vi "ex5_sharedlog.vi"() -> ()   [LabVIEW 2022 SP3]
uses:
  C:/Program Files (x86)/National Instruments/LabVIEW 2022/examples/Connectivity/Python/support/PythonVersionsEnum.ctl
  py_msg.ctl
  pylabview/pythonq.lvlib
panel:
  out "String":string
  out "xref out":string
  out "Data Out":dbl(graph)
  out "xref in":string
  in  "wait":u32=500
  out "Data IN":dbl(graph)
  in  "stop":bool
  # "https://github.com/jmor2000/labview_python_bridge"
  # "brought to you by"
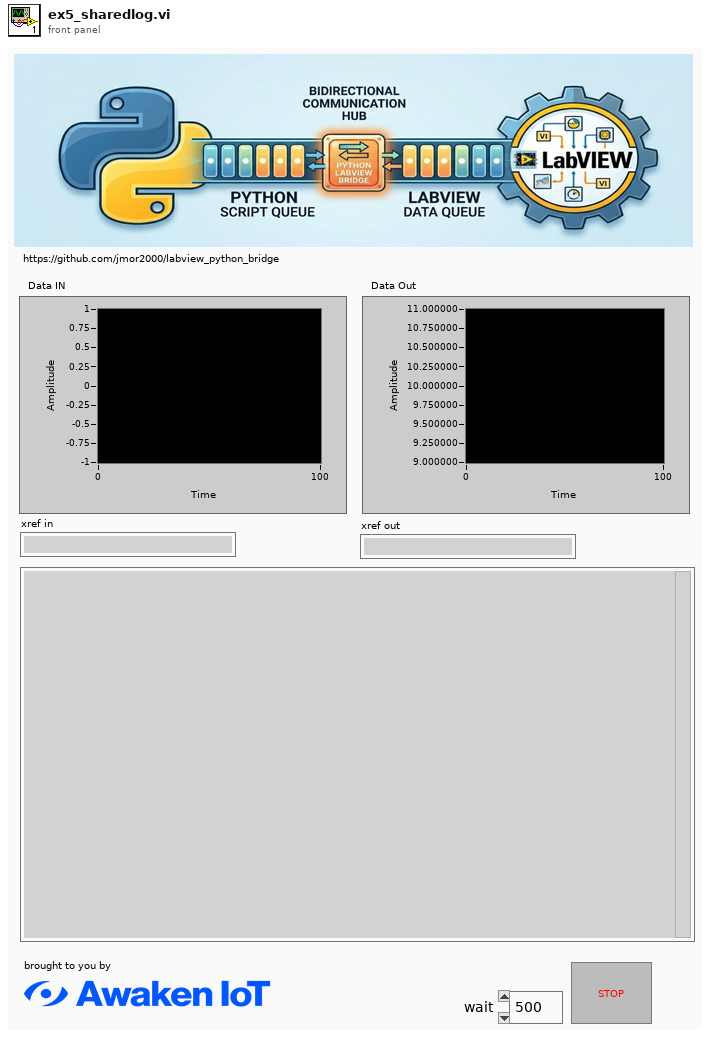
[diagram p1: front panel]
types:
  T1 = typedef "PythonVersionsEnum.ctl" = enum16{"3.6", "3.7", "3.8", "3.9"}
  T2 = typedef "pythonq.lvlib/py_cluster.ctl" = cluster{"path":path, "py":T3}
  T3 = typedef "pythonq.lvlib/py_session.ctl" = cluster{"session":refnum<k35>, "object":refnum<k38>}
  T4 = cluster{"id":string, "ts":string, "msg":string, "iref":string, "xref":string}
  T5 = typedef "pythonq.lvlib/py_result.ctl" = cluster{"value":string, "ok":bool, "error_msg":string}
  T6 = typedef "py_msg.ctl" = cluster{"double":dbl, "ref":string}
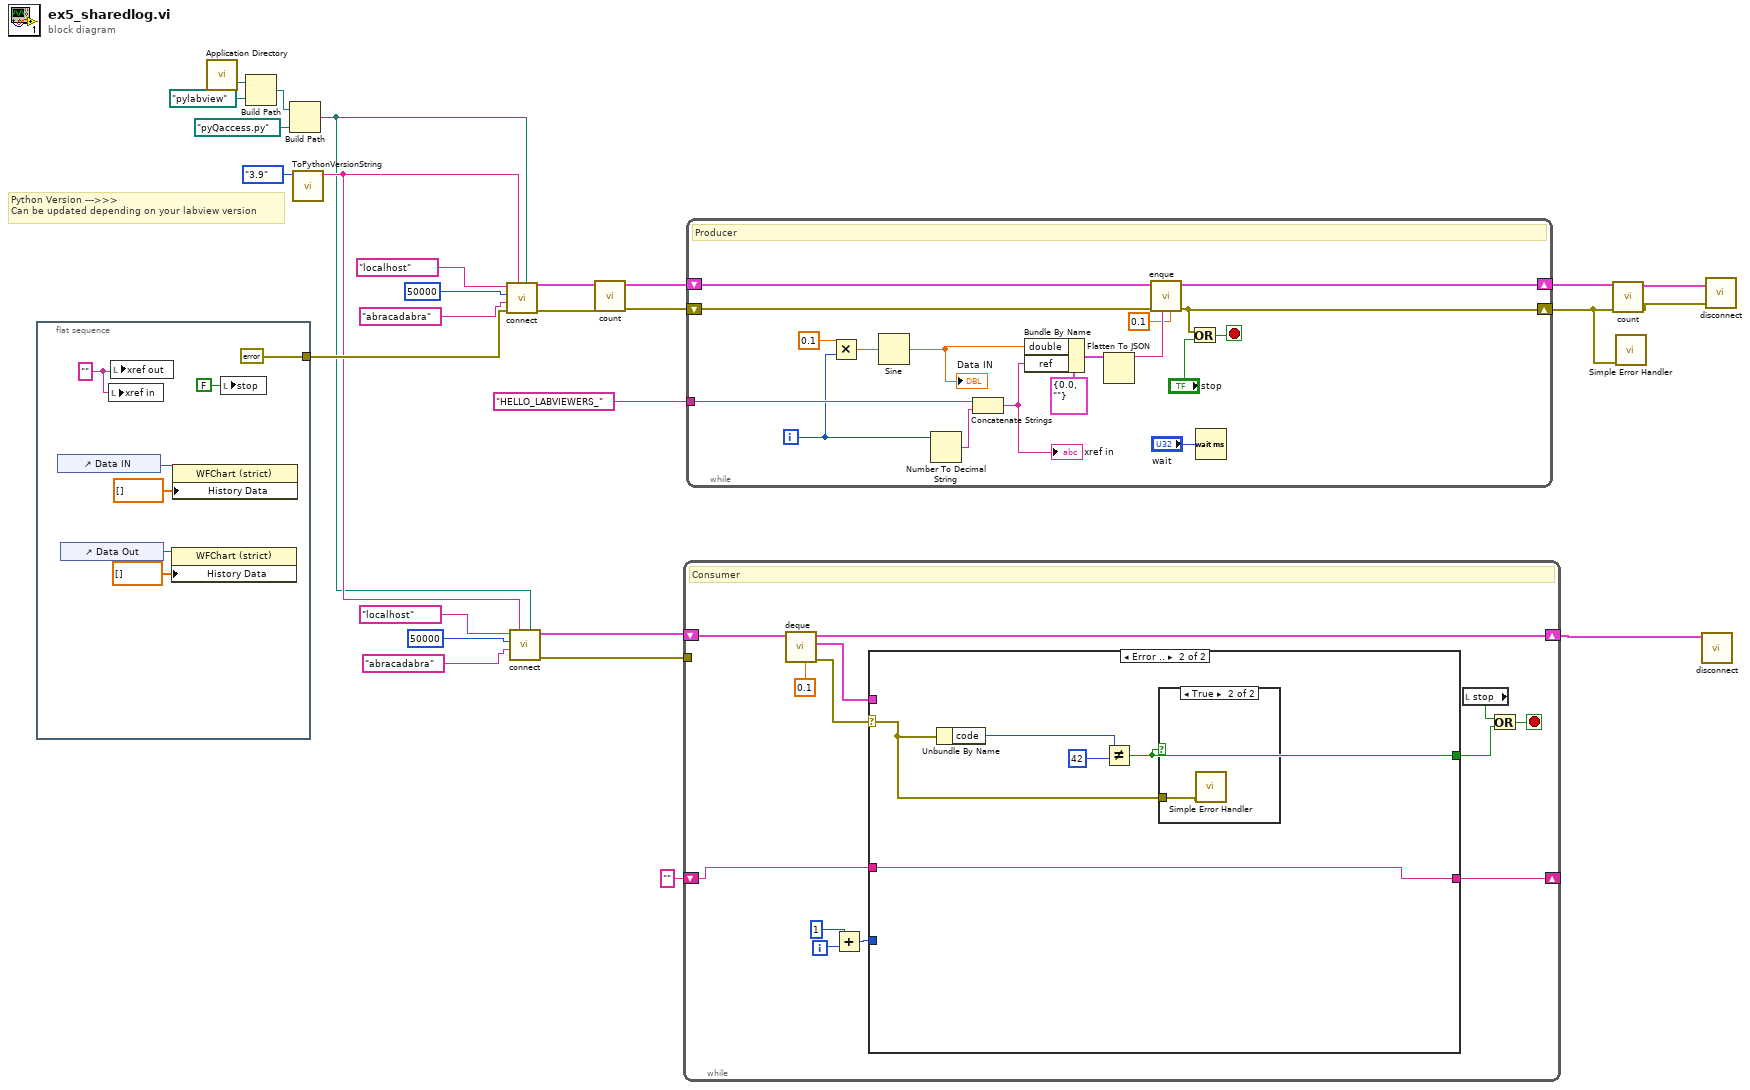
[diagram p0: block diagram]
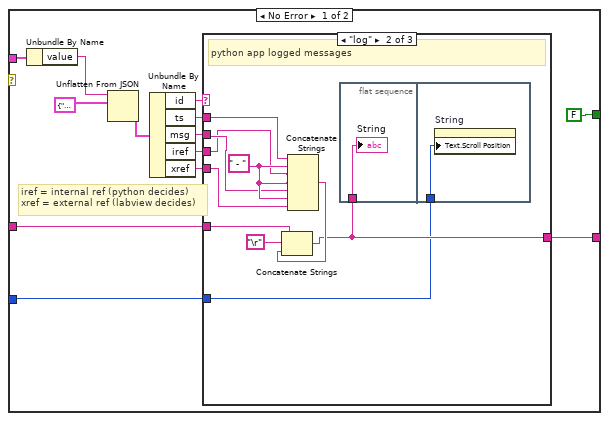
[diagram p2: hidden frame]
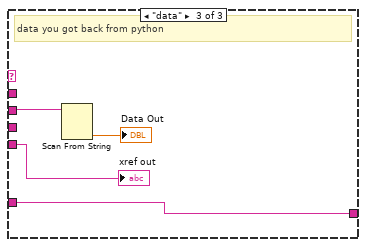
[diagram p4: hidden frame]
diagram:
  # "Python Version --->>>\nCan be updated depending on your labview version"
  n1 = flat-sequence {
    tunnel: [errorcluster {"status"=FALSE, "code"=0, "source"=""} ("error in (no error)")] -> w16
    frame #0 {
      w30 = "" ("cur ref 2")
      n2 = control-ref of="Data IN"() -> (w32:refnum<vi>)
      n3 = control-ref of="Data Out"() -> (w29:refnum<vi>)
      n4 = local write "xref in"(w30) -> ()
      n5 = local write "xref out"(w30) -> ()
      n6 = property class="WFChart (strict)"(reference=w29, "History Data"=dbl[] []) -> ()  [unwired: 1 in, 2 out]
      n7 = property class="WFChart (strict)"(reference=w32, "History Data"=dbl[] []) -> ()  [unwired: 1 in, 2 out]
      n8 = local write "stop"(FALSE ("stop")) -> ()
    }
  }
  n9 = call <vilib>:"Application Directory.vi"() -> ("Application Directory"=w22:path)
  n10 = Build Path(base path=w22, name or relative path=path "pylabview") -> (appended path=w23:path)
  n11 = Build Path(base path=w23, name or relative path=path "pyQaccess.py") -> (appended path=w7:path)
  n12 = call "ToPythonVersionString.vi"("python version"=PythonVersionsEnum."3.9") -> ("python version string"=w8:string)  [unwired: 10 in]
  n13 = call "connect.vi"("module path"=w7, "Python version"=w8, "error in (no error)"=w16, "password"="abracadabra", "port"=50000, "ip_address"="localhost") -> ("error out"=w18:errorcluster, "py out"=w17:T2)  [unwired: 4 in]
  n14 = call "connect.vi"("module path"=w7, "Python version"=w8, "password"="abracadabra", "port"=50000, "ip_address"="localhost") -> ("error out"=w5:errorcluster, "py out"=w6:T2)  [unwired: 5 in]
  n15 = call "count.vi"("error in (no error)"=w18, "py in"=w17) -> ("error out"=w15:errorcluster, "py out"=w12:T2)  [unwired: 7 in, 1 out]
  n16 = while {
    shift-right: [w46] -> w3
    shift-left: w6 -> [w47]
    tunnel: w5 -> [_]
    shift-right: [w38] -> _
    shift-left: "" -> [w39]
    i -> [w37]
    stop <- w43 stop-if-true
    # "Consumer"
    n17 = call "deque.vi"("timeout"=0.1, "py in"=w47) -> ("error out"=w44:errorcluster, "response"=w41:T5, "py out"=w46:T2)  [unwired: 6 in, 1 out]
    n18 = Add(x=1, y=w37) -> (x+y=w35:i32)
    n19 = case shown="Error .." w44 {
      selector: w44 -> [_ w78]
      tunnel: [FALSE w79] -> w42
      tunnel: w41 -> [w59 _]
      tunnel: [w50 w80] -> w38
      tunnel: w39 -> [w49 w80]
      tunnel: w35 -> [w48 _]
      frame No Error {
        # "iref = internal ref (python decides)\nxref = external ref (labview decides)"
        n20 = Unbundle By Name(w59) -> ("value"=w58:string)
        n21 = Unflatten From JSON(JSON string=w58, type and defaults=T4 {"id"="", "ts"="", "msg"="", "iref"="", "xref"=""}) -> (value=w57:T4)  [unwired: 5 in, 1 out]
        n22 = Unbundle By Name(w57) -> ("id"=w55:string, "ts"=w54:string, "msg"=w53:string, "iref"=w52:string, "xref"=w51:string)
        n23 = case shown="\"log\"" w55 {
          tunnel: w54 -> [_ w71 _]
          tunnel: w53 -> [_ w63 w77]
          tunnel: w52 -> [_ w62 _]
          tunnel: w51 -> [_ w67 w75]
          tunnel: [w61 w65 w74] -> w50
          tunnel: w49 -> [w61 w68 w74]
          tunnel: w48 -> [_ w64 _]
          frame "", Default {
            # "Unknown msg type"
          }
          frame "log" {
            w66 = " - "
            # "python app logged messages"
            n24 = Concatenate Strings(w71, w66, w62, w66, w63, w66, w67) -> (w69:string)
            n25 = Concatenate Strings(w68, "\r", w69) -> (w65:string)
            n26 = flat-sequence {
              tunnel: w65 -> [w72]
              tunnel: w64 -> [w73]
              frame #0 {
                "String" <- w72
              }
              frame #1 {
                n27 = property on="String" class="Str"("Text.Scroll Position"=w73) -> ()  [unwired: 2 in, 2 out]
              }
            }
          }
          frame "data" {
            # "data you got back from python"
            n28 = Scan From String(input string=w77) -> (output 1=→"Data Out":dbl)  [unwired: 4 in, 3 out]
            "xref out" <- w75
          }
        }
      }
      frame Error {
        n29 = Unbundle By Name(w78) -> ("code"=w82:i32)
        n30 = Not Equal?(x=w82, y=42) -> (x != y?=w79:bool)
        n31 = case shown="True" w79 {
          tunnel: w78 -> [_ w83]
          frame False {
          }
          frame True {
            n32 = call <vilib>:"Simple Error Handler.vi"("error in (no error)"=w83) -> ()  [unwired: 4 in, 5 out]
          }
        }
      }
    }
    n33 = local read "stop"() -> (w40:bool)
    n34 = Or(x=w40, y=w42) -> (x .or. y?=w43:bool)
  }
  n35 = while {
    shift-right: [w100] -> w4
    shift-left: w12 -> [w101]
    shift-right: [w97] -> w1
    shift-left: w15 -> [w99]
    tunnel: "HELLO_LABVIEWERS_" ("ref_prefix") -> [w94]
    i -> [w85]
    stop <- w98 stop-if-true
    # "Producer"
    n36 = Multiply(x=0.1, y=w85) -> (x*y=w86:dbl)
    n37 = Sine(x=w86) -> (sin(x)=w84:dbl)
    "Data IN" <- w84
    n38 = Number To Decimal String(number=w85) -> (decimal integer string=w93:string)  [unwired: 1 in]
    n39 = Concatenate Strings(w94, w93) -> (w91:string)
    "xref in" <- w91
    n40 = Bundle By Name(cluster=T6 {"double"=0.0, "ref"=""} ("Cluster"), "double"=w84, "ref"=w91) -> (w90:T6)
    n41 = Flatten To JSON(anything=w90) -> (JSON string=w89:string)  [unwired: 2 in, 1 out]
    n42 = call "enque.vi"("timeout"=0.1, "data in"=w89, "error in (no error)"=w99, "py in"=w101) -> ("error out"=w97:errorcluster, "py out"=w100:T2)  [unwired: 4 in, 2 out]
    n43 = Or(x=w97, y="stop") -> (x .or. y?=w98:bool)
    n44 = Wait (ms)(milliseconds to wait="wait") -> ()  [unwired: 1 out]
  }
  n45 = call "count.vi"("error in (no error)"=w1, "py in"=w4) -> ("error out"=w14:errorcluster, "py out"=w19:T2)  [unwired: 7 in, 1 out]
  n46 = call <vilib>:"Simple Error Handler.vi"("error in (no error)"=w1) -> ()  [unwired: 4 in, 5 out]
  n47 = call "disconnect.vi"("py in"=w3) -> ()  [unwired: 10 in, 1 out]
  n48 = call "disconnect.vi"("error in (no error)"=w14, "py in"=w19) -> ()  [unwired: 9 in, 1 out]
